vi "Write.vi"(7 "nonFull":refnum<k4>, 8 "element in":T3, 10 "parms in":T2={"subchannel"=0, "size (0)"=0, "abort (F)"=FALSE, "timeout"=-1, "ack id (0)"=0, "last elt? (F)"=FALSE, "valid? (T)"=FALSE, "GUID"=""}, 11 "messengerMbase in":refnum<class "MessengerMBase.lvclass">) -> (0 "element out":T3, 1 "wait":bool, 2 "parms out":T1, 3 "messengerMbase out":refnum<class "MessengerMBase.lvclass">)   [LabVIEW 2019, in "MessengerM.lvlib" / "MessengerMBase.lvclass"]
uses:
  <resource>/Channels/MessengerM/MessengerMBase/MessengerMBase.lvclass
  <resource>/Channels/MessengerM/Element.ctl
  <resource>/Channels/MessengerM/ParmsIn.ctl
  <resource>/Channels/MessengerM/ParmsOut.ctl
  <resource>/Channels/MessengerM/MessengerMBase/MessengerMBase.lvclass/MessengerMBase.ctl
  <resource>/Channels/MessengerM/MessengerM.lvlib
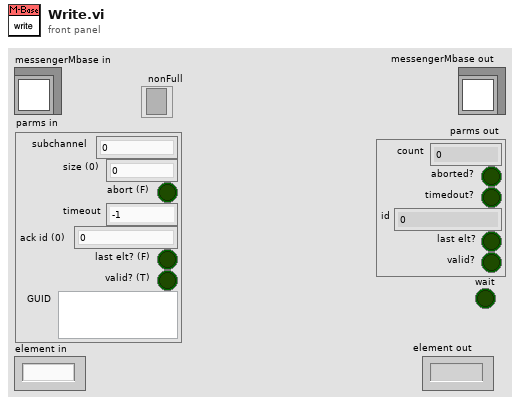
[diagram p1: front panel]
types:
  T1 = typedef "MessengerM.lvlib/ParmsOut.ctl" = cluster{"count":i32, "aborted?":bool, "timedout?":bool, "id":u32, "last elt?":bool, "valid?":bool}
  T2 = typedef "MessengerM.lvlib/ParmsIn.ctl" = cluster{"subchannel":i32, "size (0)":i32, "abort (F)":bool, "timeout":i32, "ack id (0)":u32, "last elt? (F)":bool, "valid? (T)":bool, "GUID":string}
  T3 = typedef "MessengerM.lvlib/Element.ctl" = string
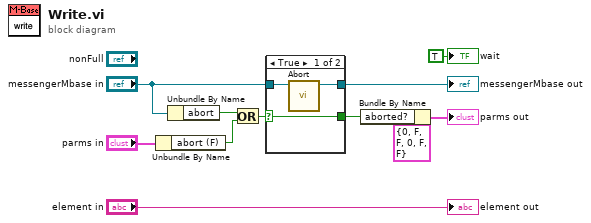
[diagram p0: block diagram]
diagram:
  n1 = Unbundle By Name("parms in") -> ("abort (F)"=w4:bool)
  n2 = Unbundle By Name("messengerMbase in") -> ("abort"=w11:bool)
  n3 = Or(x=w11, y=w4) -> (x .or. y?=w10:bool)
  n4 = case shown="True" w10 {
    selector: w10 -> [w14 _]
    tunnel: [w12 w15] -> w9
    tunnel: [w14 _] -> w3
    tunnel: "messengerMbase in" -> [w13 w15]
    frame True {
      n5 = call-dynamic "Abort.vi"("messengerMbase in"=w13) -> ("messengerMbase out"=w12:refnum<class "MessengerMBase.lvclass">)  [unwired: 10 in]
    }
    frame False {
    }
  }
  "messengerMbase out" <- w9
  n6 = Bundle By Name(cluster=T1 {"count"=0, "aborted?"=FALSE, "timedout?"=FALSE, "id"=0, "last elt?"=FALSE, "valid?"=FALSE} ("parms out"), "aborted?"=w3) -> (→"parms out":T1)
  "element out" <- "element in"
  "wait" <- TRUE ("wait")
